vi "Station Update Table For Spartan 5.0.vi"(8 "error in (no error)":errorcluster, 11 "Connection Refnum":T1) -> (0 "error out":errorcluster, 3 "Connection Refnum":T1)   [LabVIEW 2011]
uses:
  Summitek EXT/ODBC/SQL Controls/Connection Refnum.ctl
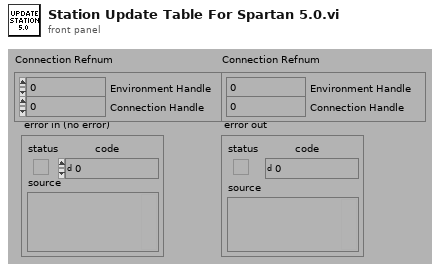
[diagram p1: front panel]
types:
  T1 = typedef "Connection Refnum.ctl" = cluster{"Environment Handle":i32, "Connection Handle":i32}
  T2 = typedef "Statement Refnum.ctl" = cluster{"Statement Handle":i32, "Parameter Number":u16}
  T3 = typedef "Association Record.ctl" = cluster{"ixAssociation":i32, "iStation":i32, "iInstrument":i32}
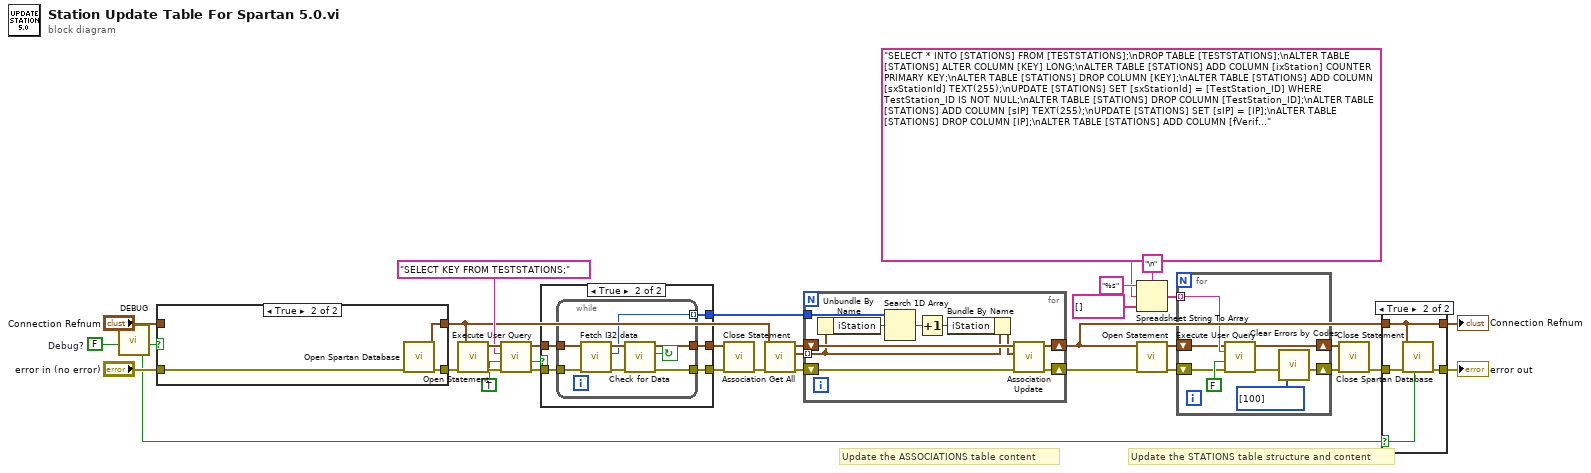
[diagram p0: block diagram]
diagram:
  w22 = FALSE  # Debug?
  # "Update the ASSOCIATIONS table content"
  # "Update the STATIONS table structure and content"
  n1 = call "DEBUG.vi"("Dev DEBUG? (f)"=w22) -> ("DEBUG?"=w21:bool)  [unwired: 1 in, 5 out]
  n2 = case shown="True" w21 {
    tunnel: "Connection Refnum" -> [w36 _]
    tunnel: "error in (no error)" -> [w35 w39]
    tunnel: [w35 w38] -> w19
    tunnel: [w36 w37] -> w7
    frame False {
    }
    frame True {
      n3 = call "Open Spartan Database.vi"("error in (no error)"=w39) -> ("error out"=w38:errorcluster, "Connection Refnum"=w37:T1)  [unwired: 2 in, 7 out]
    }
  }
  n4 = call "Open Statement.vi"("error in (no error)"=w19, "Connection Refnum"=w7) -> ("error out"=w18:errorcluster, "Statement Refnum"=w17:T2)  [unwired: 4 out]
  n5 = call "Execute User Query.vi"("error in (no error)"=w18, "Return Data? (f)"=TRUE, "User Query"="SELECT KEY FROM TESTSTATIONS;", "Statement Refnum"=w17) -> ("error out"=w14:errorcluster, "Data Present?"=w15:bool, "Statement Refnum"=w13:T2)  [unwired: 1 out]
  n6 = case shown="True" w15 {
    tunnel: w14 -> [w40 w45]
    tunnel: w13 -> [w41 w42]
    tunnel: [w40 w44] -> w12
    tunnel: [w41 w43] -> w11
    tunnel: [_ w46] -> w3
    frame False {
    }
    frame True {
      n7 = while {
        tunnel: [w51] -> w46 mode=indexing
        tunnel: w45 -> [w50]
        tunnel: [w49] -> w44
        tunnel: [w48] -> w43
        tunnel: w42 -> [w47]
        stop <- w52 continue-if-true
        n8 = call "Fetch I32 data.vi"("error in (no error)"=w50, "Statement Refnum"=w47) -> ("error out"=w54:errorcluster, "Data"=w51:i32, "Statement Refnum"=w53:T2)  [unwired: 3 out]
        n9 = call "Check for Data.vi"("error in (no error)"=w54, "Statement Refnum"=w53) -> ("error out"=w49:errorcluster, "Data Present?"=w52:bool, "Statement Refnum"=w48:T2)  [unwired: 3 out]
      }
    }
  }
  n10 = call "Close Statement.vi"("error in (no error)"=w12, "Statement Refnum"=w11) -> ("error out"=w8:errorcluster)  [unwired: 5 out]
  n11 = call "Association Get All.vi"("error in (no error)"=w8, "Connection Refnum"=w7) -> ("error out"=w6:errorcluster, "Associations"=w4:T3[], "Connection Refnum"=w5:T1)  [unwired: 7 out]
  n12 = for {
    shift-right: [w64] -> w10
    shift-left: w6 -> [w62]
    tunnel: w4 -> [w58] mode=indexing
    shift-right: [w63] -> w9
    shift-left: w5 -> [w61]
    tunnel: w3 -> [w60]
    n13 = Unbundle By Name(w58) -> ("iStation"=w59:i32)
    n14 = Search 1D Array(1D array=w60, element=w59) -> (index of element=w55:i32)  [unwired: 1 out]
    n15 = Increment(x=w55) -> (x+1=w56:i32)
    n16 = Bundle By Name(cluster=w58, "iStation"=w56) -> (w57:T3)
    n17 = call "Association Update.vi"("error in (no error)"=w62, "Association Record (empty)"=w57, "Connection Refnum"=w61) -> ("error out"=w64:errorcluster, "Connection Refnum"=w63:T1)  [unwired: 7 out]
  }
  n18 = Spreadsheet String To Array(delimiter (Tab)="\n", format string="%s", spreadsheet string="SELECT * INTO [STATIONS] FROM [TESTSTATIONS];\nDROP TABLE [TESTSTATIONS];\nALTER TABLE [STATIONS] ALTER COLUMN [KEY] LONG;\nALTER TABLE [STATIONS] ADD COLUMN [ixStation] COUNTER PRIMARY KEY;\nALTER TABLE [STATIONS] DROP COLUMN [KEY];\nALTER TABLE [STATIONS] ADD COLUMN [sxStationId] TEXT(255);\nUPDATE [STATIONS] SET [sxStationId] = [TestStation_ID] WHERE TestStation_ID IS NOT NULL;\nALTER TABLE [STATIONS] DROP COLUMN [TestStation_ID];\nALTER TABLE [STATIONS] ADD COLUMN [sIP] TEXT(255);\nUPDATE [STATIONS] SET [sIP] = [IP];\nALTER TABLE [STATIONS] DROP COLUMN [IP];\nALTER TABLE [STATIONS] ADD COLUMN [fVerified] LONG;\nUPDATE [STATIONS] SET [fVerified] = -[VERIFIED];\nALTER TABLE [STATIONS] DROP COLUMN [VERIFIED];" ("User Query"), array type (2D Dbl)=string[] []) -> (array=w33:string[])
  n19 = call "Open Statement.vi"("error in (no error)"=w10, "Connection Refnum"=w9) -> ("error out"=w30:errorcluster, "Statement Refnum"=w29:T2)  [unwired: 4 out]
  n20 = for {
    shift-right: [w65] -> w28
    shift-left: w30 -> [w69]
    tunnel: w33 -> [w71] mode=indexing
    shift-right: [w68] -> w27
    shift-left: w29 -> [w70]
    n21 = call "Execute User Query.vi"("error in (no error)"=w69, "Return Data? (f)"=FALSE, "User Query"=w71, "Statement Refnum"=w70) -> ("error out"=w66:errorcluster, "Statement Refnum"=w68:T2)  [unwired: 2 out]
    n22 = call "Clear Errors by Codes.vi"("Error Codes\nto Clear (Empty)"=i32[] [100] ("Error Codes\nto Clear (Empty)"), "error in (no error)"=w66) -> ("error out"=w65:errorcluster)  [unwired: 5 out]
  }
  n23 = call "Close Statement.vi"("error in (no error)"=w28, "Statement Refnum"=w27) -> ("error out"=w20:errorcluster)  [unwired: 5 out]
  n24 = case shown="True" w21 {
    selector: w21 -> [_ w75]
    tunnel: w20 -> [w74 w78]
    tunnel: w9 -> [w73 w76]
    tunnel: [w73 w76] -> w26
    tunnel: [w74 w77] -> w25
    frame False {
    }
    frame True {
      n25 = call "Close Spartan Database.vi"("Force Close? (f)"=w75, "error in (no error)"=w78, "Connection Refnum"=w76) -> ("error out"=w77:errorcluster)  [unwired: 2 in, 6 out]
    }
  }
  "error out" <- w25
  "Connection Refnum" <- w26
